vi "Read_Light_Team072.vi"(10 "Color Sensing Mode":string, 11 "Number of Measurements to Take":dbl) -> (3 "Average Measurement Value":dbl)   [LabVIEW 2016]
uses:
  <vilib>/NXT/Block Support/NXT_InputPort.ctl
  <vilib>/NXT/Dual Mode Library/Sensors/EV3_Color_Reflect.vi
  <vilib>/NXT/Dual Mode Library/Sensors/EV3_Color_Ambient.vi
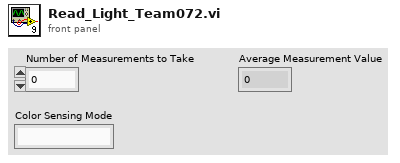
[diagram p1: front panel]
types:
  T1 = typedef "NXT_InputPort.ctl" = u32
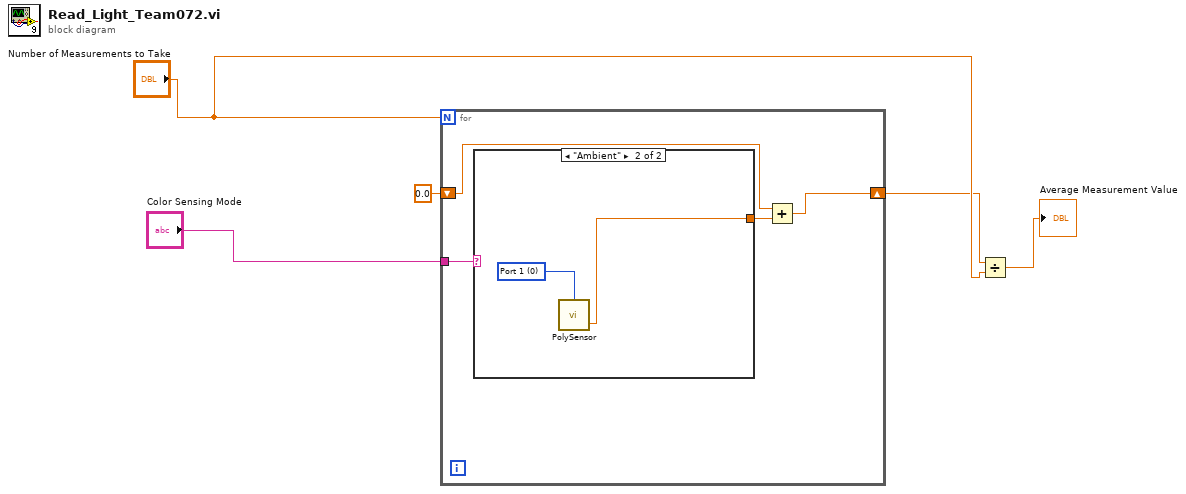
[diagram p0: block diagram]
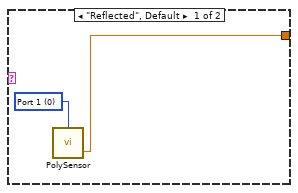
[diagram p2: hidden frame]
diagram:
  n1 = for {
    N: "Number of Measurements to Take" -> [_]
    tunnel: "Color Sensing Mode" -> [w9]
    shift-right: [w6] -> w2
    shift-left: sgl 0.0 -> [w7]
    n2 = case shown="\"Ambient\"" w9 {
      tunnel: [w11 w13] -> w8
      frame "Reflected", Default {
        w10 = T1 0 items=["Port 1", "Port 2", "Port 3", "Port 4"] ("Port (Port 1)")
        n3 = call-poly <vilib>:"PolySensor.vi"("Port (Port 1)"=w10) -> ("Scaled Value"=w11:sgl)  [unwired: 2 in, 1 out]
      }
      frame "Ambient" {
        w12 = T1 0 items=["Port 1", "Port 2", "Port 3", "Port 4"] ("Port (Port 1)")
        n4 = call-poly <vilib>:"PolySensor.vi"("Port (Port 1)"=w12) -> ("Scaled Value"=w13:sgl)  [unwired: 2 in, 1 out]
      }
    }
    n5 = Add(x=w7, y=w8) -> (x+y=w6:sgl)
  }
  n6 = Divide(x=w2, y="Number of Measurements to Take") -> (x/y=→"Average Measurement Value":dbl)
